vi "LJUD_eAddGoGet (U8 Array).vi"(0 "Handle In":i32, 1 "aIOTypes":i32[](array[numeric]), 2 "aChannels":i32[](array[numeric]), 5 "Values Write":dbl[](array[numeric]) format="%.2f", 7 "ax1s Write (U8 Arrays)":u8[][](array[numeric]), 11 "error in":errorcluster) -> (4 "Handle Out":i32, 6 "Values Read":dbl[](array[numeric]) format="%.2f", 8 "aRequestErrors":i32[](array[numeric]), 10 "GoError":i32, 13 "ax1s Read (U8 Arrays)":u8[][](array[numeric]), 14 "aResultErrors":i32[](array[numeric]), 15 "error out":errorcluster)   [LabVIEW 2021]
doc: "This is a special LabVIEW variation of eAddGoGet where each x1 is declared\nas a U8 array.\n\nThis is a call to eAddGoGet from the UD libary. By passing arrays of requests\nand results this function combines add-add-go-get-get into a single function\ncall.\n\nIn LabVIEW an alternative way to do multiple requests and results with a\nsingle sub-VI is the utility AddS-Go-Get.vi. The utility VI has better/easier\nerror handling and is normally preferred in LabVIEW, but eAddGoGet is a\nsingle call to the UD driver so often preferred if you will have parallel\ndriver calls within the same thread.\n\nThis is a traditional technique UD function ... Add-Add-Go-Get-Get. See\nSection 4.1 of the device's datasheet for more information.\n\nIOType specifies what sort of action will be performed. The other inputs\ndepend on the IOType. See the pseudocode in Section 4.3 for info."
uses:
  labjackud.dll
panel:
  # "LJUD_eAddGoGet (U8 Array).vi will likely work in 32-bit only.  If you\nneed a function like this for 64-bit contact us.  I2C is the only likely\nneed for this type of function.\n\nThis is a special LabVIEW variation of eAddGoGet where each x1 is declared\nas a U8 array.\n\nThis is a call to eAddGoGet from the UD libary.  By passing arrays of requests\nand results this function combines add-add-go-get-get into a single function\ncall.\n\nIn LabVIEW an alternative way to do multiple requests and results with a\nsingle sub-VI is the utility AddS-Go-Get.vi.  The utility VI has better/easier\nerror handling and is normally preferred in LabVIEW, but eAddGoGet is a\nsingle call to the UD driver so often preferred if you will have parallel\ndriver calls within the same thread.\n\nThis is a traditional technique UD function ... Add-Add-Go-Get-Get. See\nSection 4.1 of the device's datasheet for more information.\n\nIOType specifies what sort of action will be performed.  The other inputs\ndepend on the IOType.  See the pseudocode in Section 4.3 for info."
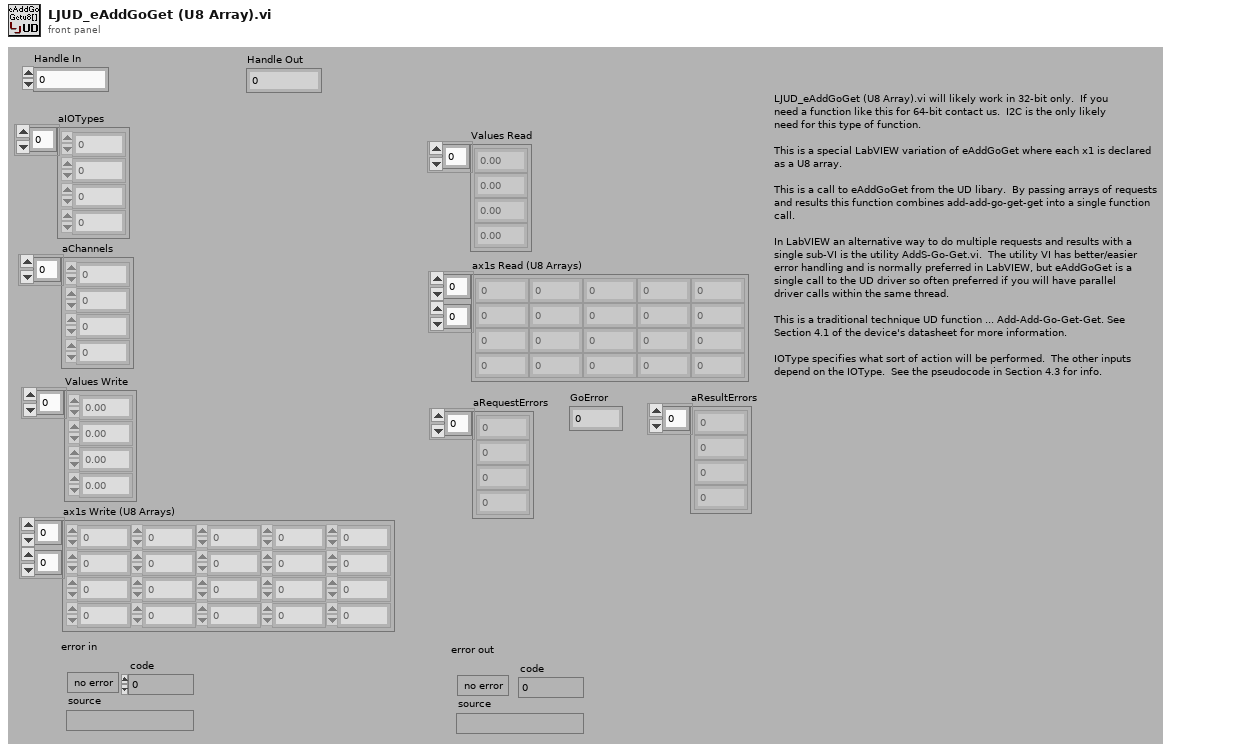
[diagram p1: front panel]
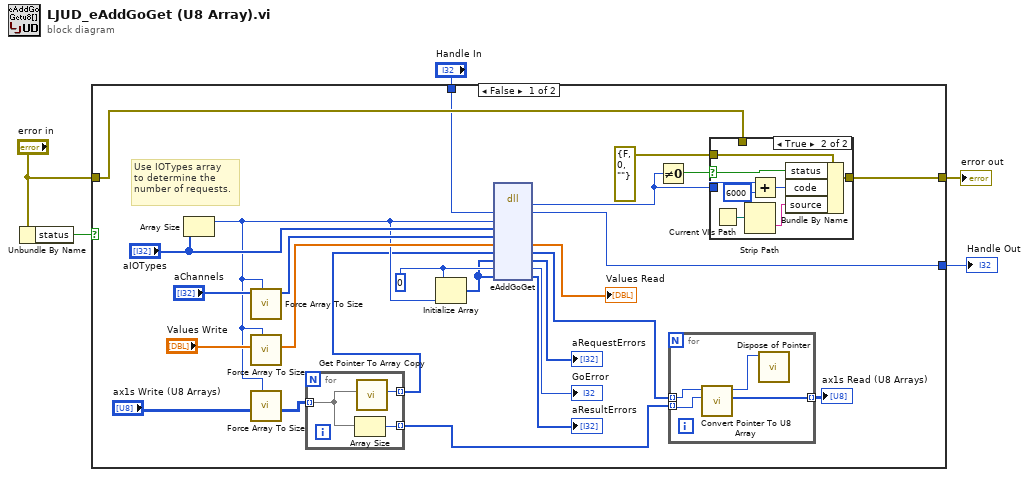
[diagram p0: block diagram]
diagram:
  n1 = Unbundle By Name("error in") -> ("status"=w4:bool)
  n2 = case shown="False" w4 {
    tunnel: [w27 w48] -> w5
    tunnel: "error in" -> [w26 w48]
    tunnel: "Handle In" -> [w19 w47]
    tunnel: [w18 w47] -> w1
    frame False {
      w25 = 0 ("GoError")
      # "Use IOTypes array\nto determine the\nnumber of requests."
      n3 = Array Size(array="aIOTypes") -> (size(s)=w12:i32)
      n4 = call "Force Array To Size.vi"("# Elements"=w12, "I32 Array In"="aChannels") -> ("I32 Array Out"=w16:i32[])  [unwired: 6 in, 3 out]
      n5 = call "Force Array To Size.vi"("# Elements"=w12, "DBL Array In"="Values Write") -> ("DBL Array Out"=w13:dbl[])  [unwired: 6 in, 3 out]
      n6 = call "Force Array To Size.vi"("# Elements"=w12, "2D U8 Array In"="ax1s Write (U8 Arrays)") -> ("2D U8 Array Out"=w10:u8[][])  [unwired: 6 in, 3 out]
      n7 = for {
        tunnel: w10 -> [w36] mode=indexing
        tunnel: [w37] -> w9 mode=indexing
        tunnel: [w35] -> w8 mode=indexing
        n8 = Array Size(array=w36) -> (size(s)=w35:i32)
        n9 = call "Get Pointer To Array Copy.vi"("U8 Array"=w36) -> ("Pointer"=w37:u32)  [unwired: 10 in]
      }
      n10 = Initialize Array(w25, w12) -> (w24:i32[])
      n11 = dll-call lib="labjackud.dll" fn="eAddGoGet"("Handle"=w19, "NumRequests"=w12, "aIOTypes"="aIOTypes", "aChannels"=w16, "aValues"=w13, "ax1s"=w9, "aRequestErrors"=w24, "GoError"=w25, "aResultErrors"=w24) -> (w28:i32, "Handle"=w18:i32, "aValues"=→"Values Read":dbl[], "ax1s"=w7:i32[], "aRequestErrors"=→"aRequestErrors":i32[], "GoError"=→"GoError":i32, "aResultErrors"=→"aResultErrors":i32[])  [unwired: 6 in, 2 out]
      n12 = Not Equal To 0?(x=w28) -> (x != 0?=w29:bool)
      n13 = for {
        tunnel: w7 -> [w32] mode=indexing
        tunnel: [w34] -> w6 mode=indexing
        tunnel: w8 -> [w33] mode=indexing
        n14 = call "Convert Pointer To U8 Array.vi"("Array Size"=w33, "Pointer"=w32) -> ("U8 Array"=w34:u8[], "Pointer Out"=w31:u32)  [unwired: 8 in]
        n15 = call "Dispose of Pointer.vi"("Pointer"=w31) -> ()  [unwired: 11 in]
      }
      "ax1s Read (U8 Arrays)" <- w6
      n16 = case shown="True" w29 {
        selector: w29 -> [_ w45]
        tunnel: [w38 w46] -> w27
        tunnel: errorcluster {"status"=FALSE, "code"=0, "source"=""} ("error IO") -> [_ w44]
        tunnel: w28 -> [_ w40]
        tunnel: w26 -> [w38 _]
        frame False {
        }
        frame True {
          n17 = Current VI's Path() -> (path=w42:path)
          n18 = Strip Path(path=w42) -> (name=w43:string)  [unwired: 1 out]
          n19 = Add(x=w40, y=6000) -> (x+y=w41:i32)
          n20 = Bundle By Name(cluster=w44, "status"=w45, "code"=w41, "source"=w43) -> (w46:errorcluster)
        }
      }
    }
    frame True {
    }
  }
  "error out" <- w5
  "Handle Out" <- w1
